vi "KVP to Variant.vi"(9 "Name":string="untitled", 10 "KVP":variant) -> (2 "Reconstructed Data":variant)   [LabVIEW 2013, in "OpenVariant.lvlib"]
doc: "This VI takes a default value as the input and replaces it recursively (cluster, array) with values found in key value pair arrays."
uses:
  OpenVariant.lvlib
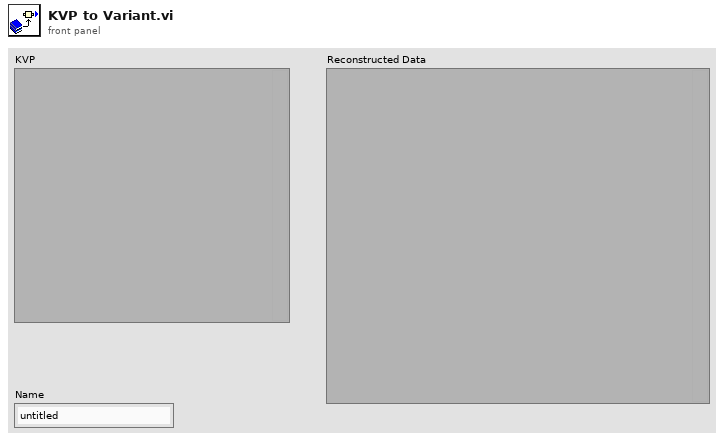
[diagram p1: front panel]
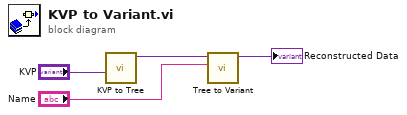
[diagram p0: block diagram]
diagram:
  n1 = call "KVP to Tree.vi"("KVP"="KVP") -> ("Variant Tree"=w3:variant)  [unwired: 10 in]
  n2 = call "Tree to Variant.vi"("Name"="Name", "Variant Tree"=w3) -> ("Variant"=→"Reconstructed Data":variant)  [unwired: 9 in]
